vi "Async Call.vi"(9 "Pour Size":string, 11 "Fill Meter Reference":refnum<vi>) -> (0 "error out":errorcluster)   [LabVIEW 2020]
panel:
  # "*Come Back* Update so it takes a VI reference?"
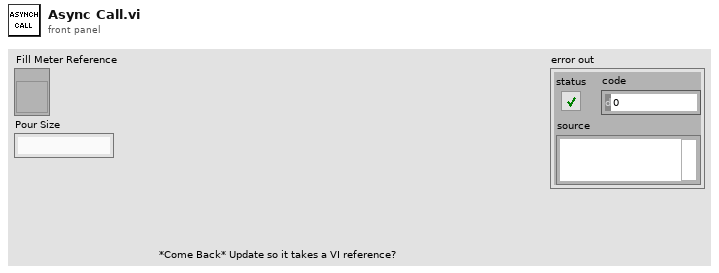
[diagram p1: front panel]
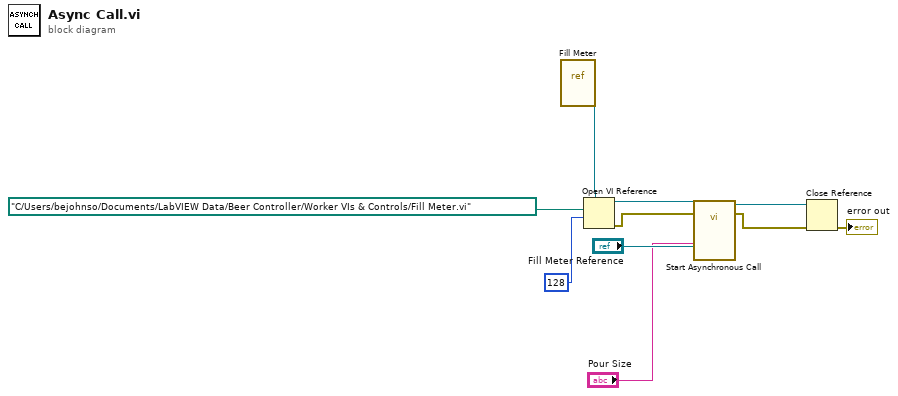
[diagram p0: block diagram]
diagram:
  n1 = vi-ref "Fill Meter.vi"() -> (w5:refnum<vi>)
  n2 = Open VI Reference(type specifier VI Refnum (for type only)=w5, vi path=path "C:/Users/bejohnso/Documents/LabVIEW Data/Beer Controller/Worker VIs & Controls/Fill Meter.vi", options=128) -> (vi reference=w1:refnum<vi>, error out=w10:errorcluster)  [unwired: 3 in]
  n3 = call-by-ref "Start Asynchronous Call"(reference=w1, error in=w10, "Pour Size"="Pour Size", "Fill Meter Reference"="Fill Meter Reference") -> (reference out=w9:refnum<vi>, error out=w8:errorcluster)  [unwired: 10 in]
  n4 = Close Reference(reference=w9, error in (no error)=w8) -> (error out=→"error out":errorcluster)
